vi "Write Eventstring and SyncPulse to Hammer.vi"(1 "error in":errorcluster, 2 "string name":string, 3 "DataSocket\nTarget":string="dstp://localhost/eventstrings") -> (0 "error out":errorcluster)   [LabVIEW 2010, in "Core SubVIs.lvlib"]
uses:
  Core SubVIs.lvlib
  <vilib>/DAQmx/write.llb/DAQmx Write (Digital Bool 1Line 1Point).vi
  <vilib>/daqmx/miscellaneous.llb/DAQmx Fill In Error Info.vi
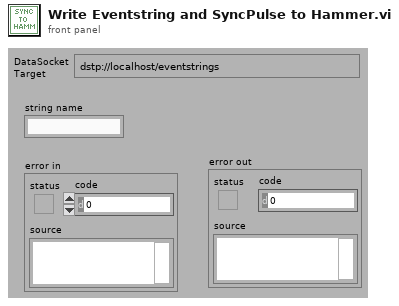
[diagram p1: front panel]
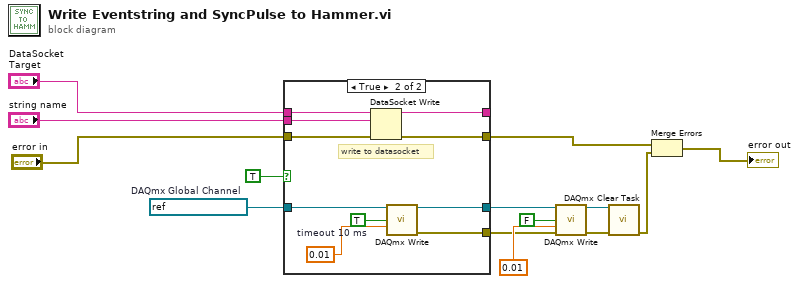
[diagram p0: block diagram]
diagram:
  w5 = refnum<k21> "EVENT_1_OUT"  # DAQmx Global Channel
  n1 = case shown="True" TRUE ("Fixated?") {
    tunnel: "error in" -> [w15 w18]
    tunnel: "DataSocket\nTarget" -> [w17 w27]
    tunnel: [w17 w26] -> _
    tunnel: [w15 w25] -> w4
    tunnel: w5 -> [w16 w22]
    tunnel: [w16 w24] -> w10
    tunnel: [w15 w23] -> w11
    tunnel: "string name" -> [_ w19]
    frame False {
      # "Data hasn't changed, so don't write to the server"
    }
    frame True {
      w21 = 0.01  # timeout 10 ms
      # "write to datasocket"
      n2 = DataSocket Write(8:w18, 10:w19, 11:w27) -> (0:w25:errorcluster, 3:w26:string)  [unwired: 1 in, 1 out]
      n3 = call-poly <vilib>:"DAQmx Write.vi"("task/channels in"=w22, "data"=TRUE ("Fixated?"), "timeout"=w21) -> ("task out"=w24:refnum<k21>, "error out"=w23:errorcluster)  [unwired: 10 in, 1 out]
    }
  }
  n4 = call-poly <vilib>:"DAQmx Write.vi"("task/channels in"=w10, "data"=FALSE ("Fixated?"), "timeout"=0.01, "error in"=w11) -> ("task out"=w13:refnum<k21>, "error out"=w12:errorcluster)  [unwired: 9 in, 1 out]
  n5 = call <vilib>:"DAQmx Clear Task.vi"("task in"=w13, "error in"=w12) -> ("error out"=w3:errorcluster)  [unwired: 13 in]
  n6 = Merge Errors(w4, w3) -> (→"error out":errorcluster)
